vi "Kinesis-Electronics-1-Old-Controllers.vi"() -> ()   [LabVIEW 2014]
doc: "André Romero - 2017\nandretec@ifsc.usp.br"
uses:
  C:/UsersLab/AndreTec/LabView2014-32bits/kinesisTec/Kinesis/Thorlabs.MotionControl.Controls.dll
  Kinesis/Thorlabs.MotionControl.Controls.dll
  Basic-VIs/motorsGlobalVar.vi
panel:
  in  "N resistors":i32=3 min=1 step=1
  in  "Adjust Motors":bool
  out "Process time":string="0:00:35"
  out "XY Graph":cluster{"Graph X":dbl[], "Graph Y":dbl[]}(graph)={"Graph X"=[0.3888467817164179, 0.38931319962686567, 0.42884211753731344, 0.6961578824626866, 1.173915578358209, 1.6747901119402986, 2.134532416044776, 2.3664004197761193, 2.388905083955224, 2.4095149253731343, 2.636864505597015, 3.09404151119403, 3.5953533115671643, 4.096315298507463, 4.5974230410447765, 5.076113572761194, 5.347014925373134, 5.38896338619403, 5.487260960820896, 5.834742304104478, 6.334625699626866, 6.835471082089552, 7.336782882462686, 7.8375116604477615, 8.237523320895523, 8.387768190298507, 8.38896338619403, 8.407241138059701, 8.629226912313433, 9.083313899253731, 9.584130130597014, 10.085471082089553, 10.586287313432836, 11.067718050373134, 11.343662546641792, 11.389079990671641, 11.407707555970148, 11.630975979477611, 12.085412779850746, 12.586578824626866, 13.087482509328359, 13.58876515858209, 14.069642024253731, 14.344362173507463, 14.389050839552239, 14.408173973880597, 14.632258628731343, 15.087045242537313, 15.588415345149254, 16.089231576492537, 16.59054337686567, 17.070720615671643, 17.344945195895523, 17.38913829291045, 17.408756996268657, 17.63368703358209, 18.089493936567163, 18.590485074626866, 19.091534514925375, 19.592933768656717, 20.072498833955223, 20.345732276119403, 20.389109141791046, 20.390391791044777, 20.54238572761194, 20.94382579291045, 21.194496268656717, 21.944350513059703, 22.14922458022388, 22.37080223880597, 22.38916744402985, 22.38916744402985], "Graph Y"=[0.26999766791044777, 0.26999766791044777, 0.26999766791044777, 0.26999766791044777, 0.26999766791044777, 0.26999766791044777, 0.26999766791044777, 0.26999766791044777, 0.26999766791044777, 0.312441697761194, 0.583809468283582, 1.0635494402985075, 1.564569729477612, 2.0656483208955225, 2.5666686100746268, 3.0233208955223883, 3.249766791044776, 3.270143423507463, 3.1355527052238807, 2.750320662313433, 2.2490088619402986, 1.748192630597015, 1.2468516791044777, 0.7457147854477612, 0.37007346082089554, 0.24498600746268656, 0.27017257462686567, 0.345703125, 0.665957322761194, 1.1609433302238805, 1.662080223880597, 2.163450326492537, 2.664208255597015, 3.0870452425373136, 3.2648087686567164, 3.2702891791044775, 3.1766266324626864, 2.834305037313433, 2.3353544776119404, 1.8342758861940298, 1.3333138992537314, 0.832147854477612, 0.41683185634328357, 0.24871735074626866, 0.27023087686567165, 0.32710471082089554, 0.6215601679104478, 1.1098122667910448, 1.6107742537313432, 2.1119111473880596, 2.612873134328358, 3.054920708955224, 3.258220615671642, 3.2703766324626864, 3.173507462686567, 2.827804337686567, 2.328358208955224, 1.8273962220149254, 1.326288479477612, 0.8253264925373134, 0.41283815298507465, 0.2482217817164179, 0.27028917910447764, 0.27028917910447764, 0.27028917910447764, 0.27028917910447764, 0.27028917910447764, 0.27028917910447764, 0.27028917910447764, 0.27028917910447764, 0.27028917910447764, 0.27028917910447764]}
  in  "Swap XY":bool
  out "stop cronometro":bool=TRUE
  in  "Stop Button":bool
  in  "Graph Y":dbl[](array[numeric])=[0.26999766791044777, 0.26999766791044777, 0.26999766791044777, 0.26999766791044777, 0.26999766791044777, 0.26999766791044777, 0.26999766791044777, 0.26999766791044777, 0.26999766791044777, 0.312441697761194, 0.583809468283582, 1.0635494402985075, 1.564569729477612, 2.0656483208955225, 2.5666686100746268, 3.0233208955223883, 3.249766791044776, 3.270143423507463, 3.1355527052238807, 2.750320662313433, 2.2490088619402986, 1.748192630597015, 1.2468516791044777, 0.7457147854477612, 0.37007346082089554, 0.24498600746268656, 0.27017257462686567, 0.345703125, 0.665957322761194, 1.1609433302238805, 1.662080223880597, 2.163450326492537, 2.664208255597015, 3.0870452425373136, 3.2648087686567164, 3.2702891791044775, 3.1766266324626864, 2.834305037313433, 2.3353544776119404, 1.8342758861940298, 1.3333138992537314, 0.832147854477612, 0.41683185634328357, 0.24871735074626866, 0.27023087686567165, 0.32710471082089554, 0.6215601679104478, 1.1098122667910448, 1.6107742537313432, 2.1119111473880596, 2.612873134328358, 3.054920708955224, 3.258220615671642, 3.2703766324626864, 3.173507462686567, 2.827804337686567, 2.328358208955224, 1.8273962220149254, 1.326288479477612, 0.8253264925373134, 0.41283815298507465, 0.2482217817164179, 0.27028917910447764, 0.27028917910447764, 0.27028917910447764, 0.27028917910447764, 0.27028917910447764, 0.27028917910447764, 0.27028917910447764, 0.27028917910447764, 0.27028917910447764, 0.27028917910447764]
  in  "Graph X":dbl[](array[numeric])=[0.3888467817164179, 0.38931319962686567, 0.42884211753731344, 0.6961578824626866, 1.173915578358209, 1.6747901119402986, 2.134532416044776, 2.3664004197761193, 2.388905083955224, 2.4095149253731343, 2.636864505597015, 3.09404151119403, 3.5953533115671643, 4.096315298507463, 4.5974230410447765, 5.076113572761194, 5.347014925373134, 5.38896338619403, 5.487260960820896, 5.834742304104478, 6.334625699626866, 6.835471082089552, 7.336782882462686, 7.8375116604477615, 8.237523320895523, 8.387768190298507, 8.38896338619403, 8.407241138059701, 8.629226912313433, 9.083313899253731, 9.584130130597014, 10.085471082089553, 10.586287313432836, 11.067718050373134, 11.343662546641792, 11.389079990671641, 11.407707555970148, 11.630975979477611, 12.085412779850746, 12.586578824626866, 13.087482509328359, 13.58876515858209, 14.069642024253731, 14.344362173507463, 14.389050839552239, 14.408173973880597, 14.632258628731343, 15.087045242537313, 15.588415345149254, 16.089231576492537, 16.59054337686567, 17.070720615671643, 17.344945195895523, 17.38913829291045, 17.408756996268657, 17.63368703358209, 18.089493936567163, 18.590485074626866, 19.091534514925375, 19.592933768656717, 20.072498833955223, 20.345732276119403, 20.389109141791046, 20.390391791044777, 20.54238572761194, 20.94382579291045, 21.194496268656717, 21.944350513059703, 22.14922458022388, 22.37080223880597, 22.38916744402985, 22.38916744402985]
  out "GetPOS Y (mm)":dbl=0.27028917910447764 format="%_6f"
  out "GetPOS X (mm)":dbl=22.38916744402985 format="%#_6f"
  out ".NET Refnum out 2":refnum<k24>
  out ".NET Refnum out 1":refnum<k24>
  out "Motor 2":bool
  out "Motor 1":bool
  in  "Acceleration (mm/s)":dbl=1.0
  in  "Iniciar":bool
  in  "Velocity (mm/s)":sgl=1.0
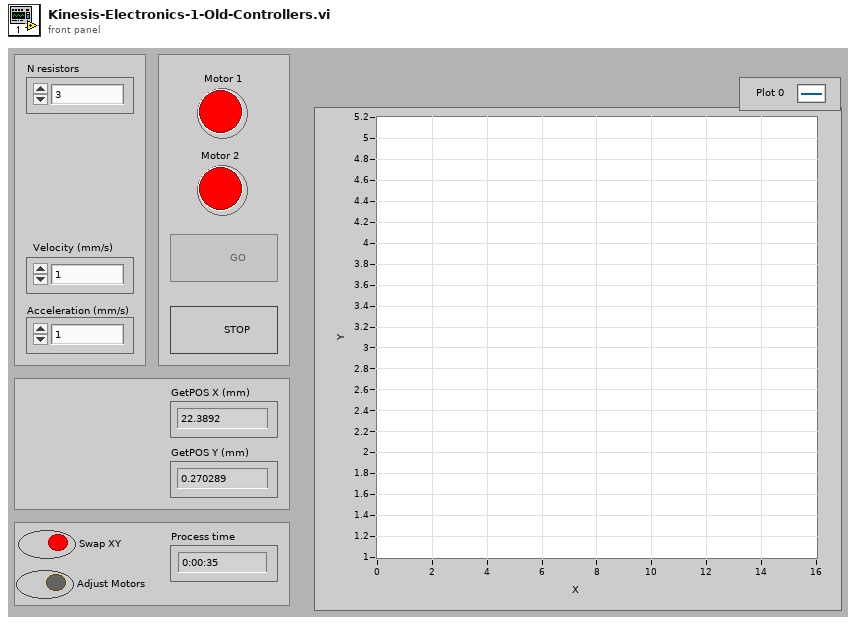
[diagram p1: front panel]
types:
  T1 = enum8{"Enabled", "Disabled", "Disabled and Grayed Out"}
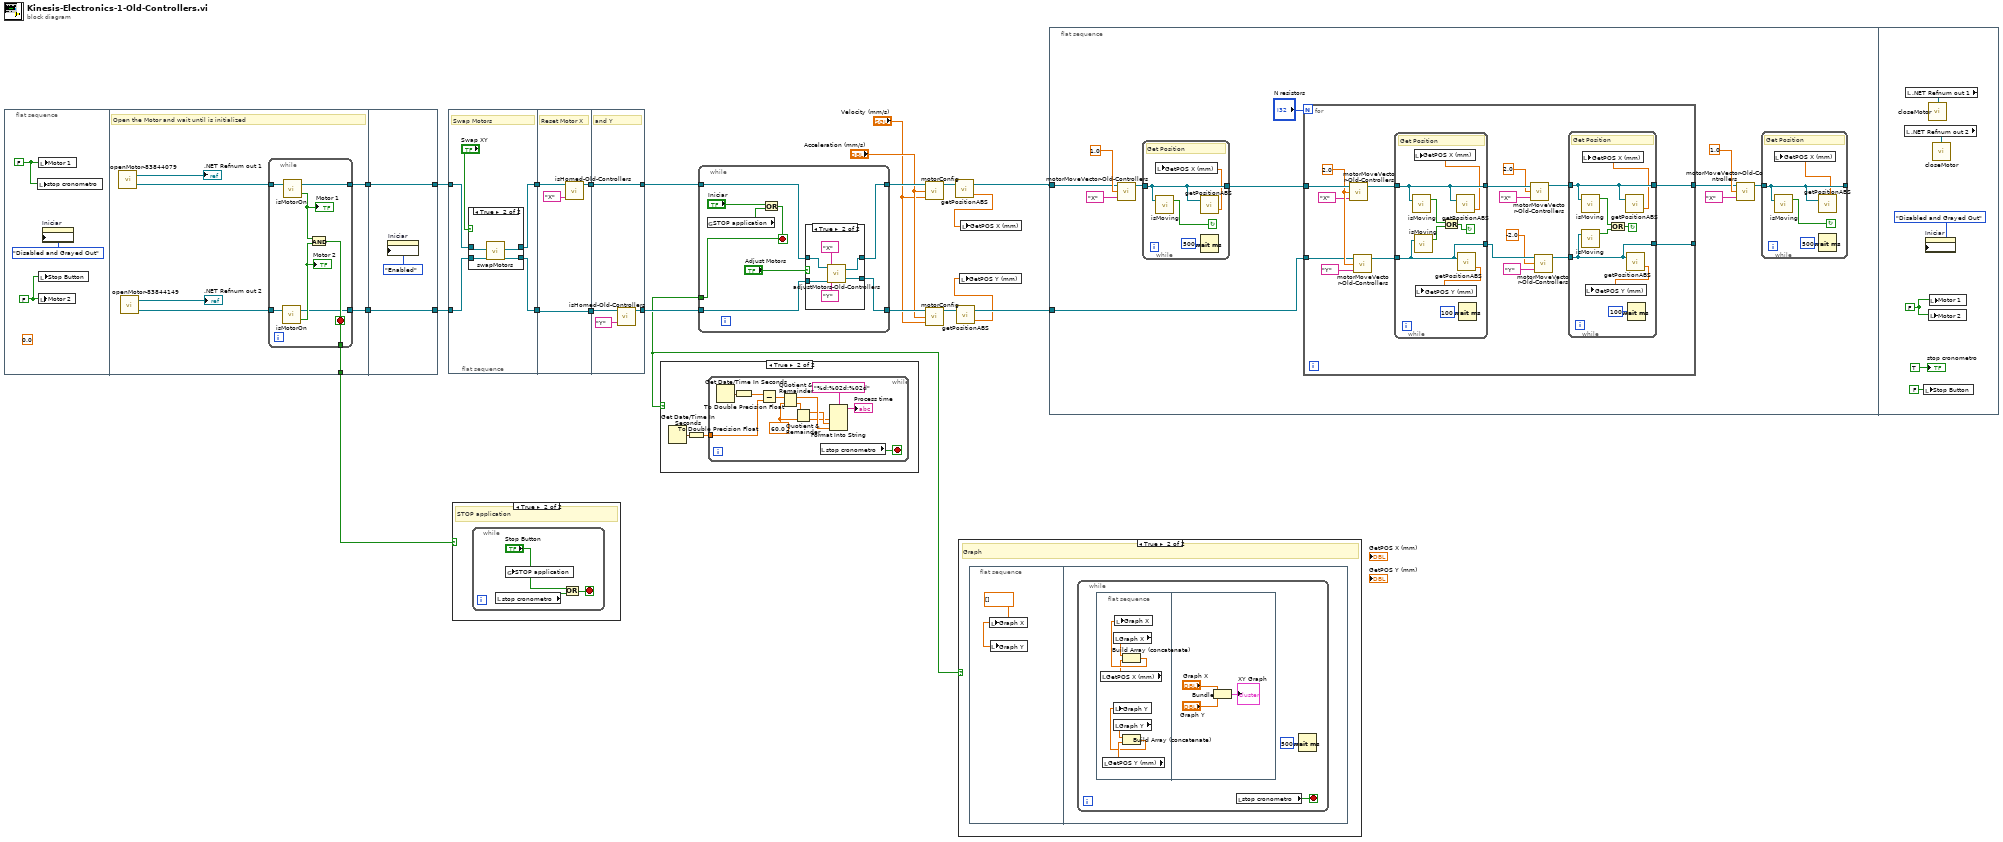
[diagram p0: block diagram]
diagram:
  n1 = flat-sequence {
    tunnel: [w28] -> w11
    tunnel: [w27] -> w10
    tunnel: [w26] -> w9
    tunnel: [w41] -> w14
    tunnel: [w42] -> w15
    tunnel: w11 -> [w42]
    tunnel: w10 -> [w41]
    frame #0 {
      (unwired) 0.0 ("Progress %")
      w24 = FALSE ("Motor3\nLigado")
      w25 = FALSE
      n2 = local write "stop cronometro"(w25) -> ()
      n3 = local write "Motor 2"(w24) -> ()
      n4 = local write "Motor 1"(w25) -> ()
      n5 = local write "Stop Button"(w24) -> ()
      n6 = property on="Iniciar" class="Bool (strict)"("DisabledEnum"=T1."Disabled and Grayed Out" ("Disabled")) -> ()  [unwired: 2 in, 2 out]
    }
    frame #1 {
      # "Open the Motor and wait until is initialized"
      n7 = call "openMotor-83844079.vi"() -> ("Device"=w30:refnum<k24>, ".NET Refnum out"=→".NET Refnum out 1":refnum<k24>)  [unwired: 2 in]
      n8 = call "openMotor-83844149.vi"() -> ("Device"=w29:refnum<k24>, ".NET Refnum out"=→".NET Refnum out 2":refnum<k24>)  [unwired: 2 in]
      n9 = while {
        tunnel: w30 -> [w37]
        tunnel: w29 -> [w36]
        tunnel: [w34] -> w28
        tunnel: [w33] -> w27
        tunnel: [w35] -> w26
        stop <- w35 stop-if-true
        n10 = call "isMotorOn.vi"("Device"=w36) -> ("isConnected"=w38:bool, "Device out"=w33:refnum<k24>)  [unwired: 1 in]
        "Motor 2" <- w38
        n11 = call "isMotorOn.vi"("Device"=w37) -> ("isConnected"=w39:bool, "Device out"=w34:refnum<k24>)  [unwired: 1 in]
        "Motor 1" <- w39
        n12 = And(x=w39, y=w38) -> (x .and. y?=w35:bool)
      }
    }
    frame #2 {
      n13 = property on="Iniciar" class="Bool (strict)"("DisabledEnum"=T1."Enabled" ("Disabled")) -> ()  [unwired: 2 in, 2 out]
    }
  }
  n14 = flat-sequence {
    tunnel: w14 -> [w46]
    tunnel: w15 -> [w47]
    tunnel: [w45] -> w8
    tunnel: [w44] -> w7
    tunnel: [w54] -> w13
    tunnel: [w57] -> w12
    tunnel: w8 -> [w55]
    tunnel: w7 -> [w57]
    tunnel: [w61] -> w18
    tunnel: [w59] -> w17
    tunnel: w13 -> [w61]
    tunnel: w12 -> [w58]
    frame #0 {
      # "Swap Motors"
      n15 = case shown="True" "Swap XY" {
        tunnel: w47 -> [w49 w53]
        tunnel: w46 -> [w48 w52]
        tunnel: [w49 w51] -> w45
        tunnel: [w48 w50] -> w44
        frame False {
        }
        frame True {
          n16 = call "swapMotors.vi"("Device 2"=w52, "Device 1"=w53) -> ("Device out 1"=w50:refnum<k24>, "Device out 2"=w51:refnum<k24>)  [unwired: 2 in, 2 out]
        }
      }
    }
    frame #1 {
      # "Reset Motor X"
      n17 = call "isHomed-Old-Controllers.vi"("Motor (XYZ)"="X", "Device in"=w55) -> ("Device out"=w54:refnum<k24>)  [unwired: 3 in]
    }
    frame #2 {
      # "and Y"
      n18 = call "isHomed-Old-Controllers.vi"("Motor (XYZ)"="Y", "Device in"=w58) -> ("Device out"=w59:refnum<k24>)  [unwired: 3 in]
    }
  }
  n19 = case shown="True" w9 {
    frame False {
    }
    frame True {
      # "STOP application"
      n20 = while {
        stop <- w63 stop-if-true
        n21 = local read "stop cronometro"() -> (w62:bool)
        n22 = global write "motorsGlobalVar.vi" "STOP application"("Stop Button") -> ()
        n23 = Or(x="Stop Button", y=w62) -> (x .or. y?=w63:bool)
      }
    }
  }
  n24 = while {
    tunnel: [w70] -> w16
    tunnel: w18 -> [w67]
    tunnel: w17 -> [w68]
    tunnel: [w66] -> w22
    tunnel: [w65] -> w21
    stop <- w70 stop-if-true
    n25 = global read "motorsGlobalVar.vi" "STOP application"() -> (w71:bool)
    n26 = Or(x="Iniciar", y=w71) -> (x .or. y?=w70:bool)
    n27 = case shown="True" "Adjust Motors" {
      tunnel: w67 -> [w74 w80]
      tunnel: w68 -> [w73 w79]
      tunnel: [w74 w78] -> w66
      tunnel: [w73 w77] -> w65
      frame False {
      }
      frame True {
        n28 = call "adjustMotors-Old-Controllers.vi"("Device 2"=w79, "Motor Y"="Y", "Motor X"="X", "Device 1"=w80) -> ("Device out 2"=w77:refnum<k24>, "Device out 1"=w78:refnum<k24>)
      }
    }
  }
  n29 = case shown="True" w16 {
    frame False {
    }
    frame True {
      n30 = Get Date/Time In Seconds() -> (seconds since 1Jan1904=w82:timestamp)
      n31 = To Double Precision Float(number=w82) -> (double precision float=w81:dbl)
      n32 = while {
        tunnel: w81 -> [w86]
        stop <- w94 stop-if-true
        w91 = 60.0 ("y")
        n33 = Get Date/Time In Seconds() -> (seconds since 1Jan1904=w93:timestamp)
        n34 = To Double Precision Float(number=w93) -> (double precision float=w87:dbl)
        n35 = Subtract(x=w87, y=w86) -> (x-y=w85:dbl)
        n36 = Quotient & Remainder(x=w85, y=w91) -> (x-y*floor(x/y)=w90:dbl, floor(x/y)=w92:dbl)
        n37 = Quotient & Remainder(x=w92, y=w91) -> (x-y*floor(x/y)=w89:dbl, floor(x/y)=w88:dbl)
        n38 = local read "stop cronometro"() -> (w94:bool)
        n39 = Format Into String(format string="%d:%02d:%02d", w88, w89, w90) -> (resulting string=→"Process time":string)  [unwired: 2 in, 1 out]
      }
    }
  }
  n40 = call "motorConfig.vi"("Velocity"="Velocity (mm/s)", "Acceleration"="Acceleration (mm/s)", "Device in"=w22) -> ("Device out"=w6:refnum<k24>)  [unwired: 2 in]
  n41 = call "motorConfig.vi"("Velocity"="Velocity (mm/s)", "Acceleration"="Acceleration (mm/s)", "Device in"=w21) -> ("Device out"=w5:refnum<k24>)  [unwired: 2 in]
  n42 = call "getPositionABS.vi"("Device"=w6) -> ("GetPOS"=w2:dbl, "Device out"=w1:refnum<k24>)  [unwired: 1 in]
  n43 = call "getPositionABS.vi"("Device"=w5) -> ("GetPOS"=w3:dbl, "Device out"=w4:refnum<k24>)  [unwired: 1 in]
  n44 = case shown="True" w16 {
    frame False {
    }
    frame True {
      # "Graph"
      n45 = flat-sequence {
        frame #0 {
          w95 = dbl[] [] ("Graph Y")
          n46 = local write "Graph X"(w95) -> ()
          n47 = local write "Graph Y"(w95) -> ()
        }
        frame #1 {
          n48 = while {
            stop <- w96 stop-if-true
            n49 = flat-sequence {
              frame #0 {
                n50 = local read "GetPOS X (mm)"() -> (w101:dbl)
                n51 = local read "GetPOS Y (mm)"() -> (w100:dbl)
                n52 = local read "Graph X"() -> (w103:dbl[])
                n53 = local read "Graph Y"() -> (w98:dbl[])
                n54 = Build Array (concatenate)(w103, w101) -> (w102:dbl[])
                n55 = local write "Graph X"(w102) -> ()
                n56 = Build Array (concatenate)(w98, w100) -> (w99:dbl[])
                n57 = local write "Graph Y"(w99) -> ()
              }
              frame #1 {
                n58 = Bundle("Graph X"="Graph X", "Graph Y"="Graph Y") -> (→"XY Graph":cluster{"Graph X":dbl[], "Graph Y":dbl[]})  [unwired: 1 in]
              }
            }
            n59 = local read "stop cronometro"() -> (w96:bool)
            n60 = Wait (ms)(milliseconds to wait=u32 500) -> ()  [unwired: 1 out]
          }
        }
      }
    }
  }
  n61 = local write "GetPOS Y (mm)"(w3) -> ()
  n62 = local write "GetPOS X (mm)"(w2) -> ()
  n63 = flat-sequence {
    tunnel: w4 -> [w117]
    tunnel: w1 -> [w108]
    frame #0 {
      n64 = call "motorMoveVector-Old-Controllers.vi"("Motor (XYZ)"="X", "Distance"=1.0 ("position"), "Device in"=w108) -> ("Device out"=w111:refnum<k24>)  [unwired: 2 in]
      n65 = while {
        tunnel: w111 -> [w121]
        tunnel: [w121] -> w107
        stop <- w120 continue-if-true
        # "Get Position"
        n66 = call "isMoving.vi"("Device in"=w121) -> ("IsMoving"=w120:bool)  [unwired: 2 in]
        n67 = call "getPositionABS.vi"("Device"=w121) -> ("GetPOS"=w118:dbl)  [unwired: 1 in, 1 out]
        n68 = local write "GetPOS X (mm)"(w118) -> ()
        n69 = Wait (ms)(milliseconds to wait=u32 500) -> ()  [unwired: 1 out]
      }
      n70 = for {
        N: "N resistors" -> [_]
        tunnel: w107 -> [w140]
        tunnel: w117 -> [w138]
        tunnel: [w127] -> w112
        tunnel: [w126] -> _
        w139 = 2.0 ("position")
        n71 = call "motorMoveVector-Old-Controllers.vi"("Motor (XYZ)"="X", "Distance"=w139, "Device in"=w140) -> ("Device out"=w142:refnum<k24>)  [unwired: 2 in]
        n72 = call "motorMoveVector-Old-Controllers.vi"("Motor (XYZ)"="Y", "Distance"=w139, "Device in"=w138) -> ("Device out"=w141:refnum<k24>)  [unwired: 2 in]
        n73 = while {
          tunnel: w142 -> [w158]
          tunnel: [w158] -> w136
          tunnel: w141 -> [w154]
          tunnel: [w154] -> w137
          stop <- w151 continue-if-true
          # "Get Position"
          n74 = call "isMoving.vi"("Device in"=w158) -> ("IsMoving"=w152:bool)  [unwired: 2 in]
          n75 = call "isMoving.vi"("Device in"=w154) -> ("IsMoving"=w153:bool)  [unwired: 2 in]
          n76 = Or(x=w152, y=w153) -> (x .or. y?=w151:bool)
          n77 = call "getPositionABS.vi"("Device"=w158) -> ("GetPOS"=w156:dbl)  [unwired: 1 in, 1 out]
          n78 = local write "GetPOS X (mm)"(w156) -> ()
          n79 = call "getPositionABS.vi"("Device"=w154) -> ("GetPOS"=w157:dbl)  [unwired: 1 in, 1 out]
          n80 = local write "GetPOS Y (mm)"(w157) -> ()
          n81 = Wait (ms)(milliseconds to wait=u32 100) -> ()  [unwired: 1 out]
        }
        n82 = call "motorMoveVector-Old-Controllers.vi"("Motor (XYZ)"="X", "Distance"=2.0 ("position"), "Device in"=w136) -> ("Device out"=w135:refnum<k24>)  [unwired: 2 in]
        n83 = call "motorMoveVector-Old-Controllers.vi"("Motor (XYZ)"="Y", "Distance"=sgl -2.0, "Device in"=w137) -> ("Device out"=w134:refnum<k24>)  [unwired: 2 in]
        n84 = while {
          tunnel: w135 -> [w150]
          tunnel: [w150] -> w127
          tunnel: w134 -> [w143]
          tunnel: [w143] -> w126
          stop <- w146 continue-if-true
          # "Get Position"
          n85 = call "isMoving.vi"("Device in"=w150) -> ("IsMoving"=w145:bool)  [unwired: 2 in]
          n86 = call "isMoving.vi"("Device in"=w143) -> ("IsMoving"=w144:bool)  [unwired: 2 in]
          n87 = Or(x=w145, y=w144) -> (x .or. y?=w146:bool)
          n88 = call "getPositionABS.vi"("Device"=w150) -> ("GetPOS"=w148:dbl)  [unwired: 1 in, 1 out]
          n89 = local write "GetPOS X (mm)"(w148) -> ()
          n90 = call "getPositionABS.vi"("Device"=w143) -> ("GetPOS"=w147:dbl)  [unwired: 1 in, 1 out]
          n91 = local write "GetPOS Y (mm)"(w147) -> ()
          n92 = Wait (ms)(milliseconds to wait=u32 100) -> ()  [unwired: 1 out]
        }
      }
      n93 = call "motorMoveVector-Old-Controllers.vi"("Motor (XYZ)"="X", "Distance"=1.0 ("position"), "Device in"=w112) -> ("Device out"=w115:refnum<k24>)  [unwired: 2 in]
      n94 = while {
        tunnel: w115 -> [w125]
        tunnel: [w125] -> _
        stop <- w124 continue-if-true
        # "Get Position"
        n95 = call "isMoving.vi"("Device in"=w125) -> ("IsMoving"=w124:bool)  [unwired: 2 in]
        n96 = call "getPositionABS.vi"("Device"=w125) -> ("GetPOS"=w122:dbl)  [unwired: 1 in, 1 out]
        n97 = local write "GetPOS X (mm)"(w122) -> ()
        n98 = Wait (ms)(milliseconds to wait=u32 500) -> ()  [unwired: 1 out]
      }
    }
    frame #1 {
      w162 = FALSE
      n99 = local read ".NET Refnum out 2"() -> (w163:refnum<k24>)
      n100 = local read ".NET Refnum out 1"() -> (w164:refnum<k24>)
      n101 = local write "Stop Button"(FALSE ("Stop Button")) -> ()
      n102 = property on="Iniciar" class="Bool (strict)"("DisabledEnum"=T1."Disabled and Grayed Out" ("Disabled")) -> ()  [unwired: 2 in, 2 out]
      n103 = call "closeMotor.vi"(".NET Refnum in"=w164) -> ()  [unwired: 2 in]
      n104 = local write "Motor 2"(w162) -> ()
      n105 = local write "Motor 1"(w162) -> ()
      n106 = call "closeMotor.vi"(".NET Refnum in"=w163) -> ()  [unwired: 2 in]
      "stop cronometro" <- TRUE ("stop cronometro")
    }
  }
